vi "LSMcontroller_v57.vi"() -> ()   [LabVIEW 2015] (continued)
                              }
                            }
                          }
                        }
                        frame True {
                        }
                      }
                      n2928 = local read "sealtest 2"() -> (w5970:bool)
                      n2929 = Not(x=w5970) -> (.not. x?=w5969:bool)
                    }
                  }
                  frame #4 {
                    n2930 = call "tempconfigAO.vi"("command"="get") -> ("Temp Config out"=w6140:T27)  [unwired: 1 in]
                    n2931 = Unbundle By Name(w6140) -> ("AO"=w6139:refnum<k21>[], "E_AO"=w6138:errorcluster[])
                    n2932 = call "configuration.vi"("command"="get") -> ("config out"=w6121:T13)  [unwired: 2 in, 1 out]
                    n2933 = call "tempconfigAI.vi"("command"="get") -> ("Temp Config out"=w6127:T28)  [unwired: 1 in]
                    n2934 = Unbundle By Name(w6121) -> ("Device 1 sampleclock out"=w6118:tag, "Device 1 Starttrigger out"=w6117:tag)
                    n2935 = Unbundle By Name(w6127) -> ("AI"=w6128:refnum<k21>, "E_AI"=w6129:errorcluster)
                    n2936 = for {
                      tunnel: w6139 -> [w6144] mode=indexing
                      tunnel: w6138 -> [w6143] mode=indexing
                      tunnel: [w6142] -> w6134 mode=indexing
                      n2937 = call <vilib>:"DAQmx Stop Task.vi"("task/channels in"=w6144, "error in"=w6143) -> ("task out"=w6145:refnum<k21>, "error out"=w6146:errorcluster)  [unwired: 12 in]
                      n2938 = call <vilib>:"DAQmx Clear Task.vi"("task in"=w6145, "error in"=w6146) -> ("error out"=w6142:errorcluster)  [unwired: 13 in]
                    }
                    n2939 = call <vilib>:"DAQmx Stop Task.vi"("task/channels in"=w6128, "error in"=w6129) -> ("task out"=w6125:refnum<k21>, "error out"=w6124:errorcluster)  [unwired: 12 in]
                    n2940 = call <vilib>:"DAQmx Disconnect Terminals.vi"("source terminal"=tag "/Dev1/ai/SampleClock", "destination terminal"=w6118) -> ("error out"=w6115:errorcluster)  [unwired: 13 in]
                    n2941 = call <vilib>:"DAQmx Clear Task.vi"("task in"=w6125, "error in"=w6124) -> ("error out"=w6123:errorcluster)  [unwired: 13 in]
                    n2942 = call "tempconfigAO.vi"("command"="get") -> ("Temp Config out"=w6135:T27)  [unwired: 1 in]
                    n2943 = Bundle By Name(cluster=w6135, "E_AO"=w6134) -> (w6133:T27)
                    n2944 = call "tempconfigAI.vi"("command"="get") -> ("Temp Config out"=w6131:T28)  [unwired: 1 in]
                    n2945 = Bundle By Name(cluster=w6131, "E_AI"=w6123) -> (w6122:T28)
                    n2946 = call "tempconfigAO.vi"("Temp Config in"=w6133, "command"="set") -> ()  [unwired: 1 out]
                    n2947 = call <vilib>:"DAQmx Disconnect Terminals.vi"("source terminal"=tag "/Dev1/ai/StartTrigger", "destination terminal"=w6117, "error in"=w6115) -> ()  [unwired: 12 in, 1 out]
                    n2948 = call "tempconfigAI.vi"("Temp Config in"=w6122, "command"="set") -> ()  [unwired: 1 out]
                  }
                  frame #5 {
                    w6149 = T23 4 items=["no dialog", "OK message", "continue or stop message", "OK message + warnings", "continue/stop + warnings"] ("type of dialog (OK msg:1)")
                    n2949 = call "displayerrors.vi"() -> ("error IO"=w6148:errorcluster)
                    n2950 = call "zeropatch.vi"() -> ()  [unwired: 12 in]
                    n2951 = call <vilib>:"Simple Error Handler.vi"("type of dialog (OK msg:1)"=w6149, "error in (no error)"=w6148) -> ("error out"=w6147:errorcluster)  [unwired: 3 in, 4 out]
                    n2952 = call <vilib>:"Clear Errors.vi"("error in (no error)"=w6147) -> ()  [unwired: 5 in, 2 out]
                  }
                }
              }
            }
          }
          event "Current Clamp": Value Change {
            n2953 = event-data() -> ()  [unwired: 1 in, 6 out]
            n2954 = local read "Current Clamp"() -> (w6154:bool)
            n2955 = property on="Vholding (mV)" class="DigNum (strict)"("Caption.Text"="Ihold (pA)") -> ()  [unwired: 2 in, 2 out]
            n2956 = Not(x=w6154) -> (.not. x?=w6153:bool)
            n2957 = property on="Voltage Clamp" class="Bool (strict)"("Value"=w6153) -> ()  [unwired: 2 in, 2 out]
            n2958 = One Button Dialog(message="Have you switched the HEKA to CC and changed the external input cable?", button name ("OK")="Ok") -> ()  [unwired: 1 out]
          }
          event "Voltage Clamp": Value Change {
            n2959 = event-data() -> ()  [unwired: 1 in, 6 out]
            n2960 = local read "Voltage Clamp"() -> (w6159:bool)
            n2961 = Not(x=w6159) -> (.not. x?=w6158:bool)
            n2962 = property on="Current Clamp" class="Bool (strict)"("Value"=w6158) -> ()  [unwired: 2 in, 2 out]
            n2963 = One Button Dialog(message="Have you switched the HEKA to VC and changed the external input cable?", button name ("OK")="Ok") -> ()  [unwired: 1 out]
            n2964 = property on="Vholding (mV)" class="DigNum (strict)"("Caption.Text"="Vhold (mV)") -> ()  [unwired: 2 in, 2 out]
          }
          event "OCgain": Value Change {
            n2965 = event-data() -> ()  [unwired: 1 in, 6 out]
            n2966 = local read "OCgain"() -> (w6162:sgl)
            n2967 = Less?(x=w6162, y=0.3) -> (x < y?=w6160:bool)
            n2968 = case shown="True" w6160 {
              frame False {
                w6163 = 10.0 items=["0.1"=10.0, "10"=0.1] ("CC_ICgain")
                n2969 = local write "CC_ICgain"(w6163) -> ()
              }
              frame True {
                w6164 = 0.1 items=["0.1"=10.0, "10"=0.1] ("CC_ICgain")
                n2970 = local write "CC_ICgain"(w6164) -> ()
              }
            }
          }
          event "holdon": Value Change {
            n2971 = event-data() -> ()  [unwired: 1 in, 6 out]
            n2972 = stacked-sequence {
              frame #0 {
                n2973 = local read "Vholding (mV)"() -> (w6168:sgl)
                n2974 = local read "holdon"() -> (w6165:bool)
                n2975 = call "patchparameters.vi"("command"="get") -> ("Params out"=w6169:T15)  [unwired: 1 in]
                n2976 = Bundle By Name(cluster=w6169, "Vhold (mV)"=w6168, "holdon"=w6165) -> (w6166:T15)
                n2977 = call "patchparameters.vi"("Params in"=w6166, "command"="set") -> ()  [unwired: 1 out]
              }
              frame #1 {
                n2978 = call "zeropatch.vi"() -> ()  [unwired: 12 in]
              }
            }
          }
          event "Vholding (mV)": Value Change {
            n2979 = event-data() -> ()  [unwired: 1 in, 6 out]
            n2980 = local read "holdon"() -> (w6171:bool)
            n2981 = case shown="True" w6171 {
              frame False {
              }
              frame True {
                n2982 = stacked-sequence {
                  frame #0 {
                    n2983 = local read "Vholding (mV)"() -> (w6174:sgl)
                    n2984 = local read "holdon"() -> (w6175:bool)
                    n2985 = call "patchparameters.vi"("command"="get") -> ("Params out"=w6176:T15)  [unwired: 1 in]
                    n2986 = Bundle By Name(cluster=w6176, "Vhold (mV)"=w6174, "holdon"=w6175) -> (w6172:T15)
                    n2987 = call "patchparameters.vi"("Params in"=w6172, "command"="set") -> ()  [unwired: 1 out]
                  }
                  frame #1 {
                    n2988 = call "zeropatch.vi"() -> ()  [unwired: 12 in]
                  }
                }
              }
            }
          }
          event "readpatch": Value Change {
            n2989 = event-data() -> ("NewVal"=w6178:bool)  [unwired: 1 in, 5 out]
            n2990 = case shown="True" w6178 {
              frame False {
              }
              frame True {
                n2991 = stacked-sequence {
                  frame #0 {
                    n2992 = stacked-sequence {
                      frame #0 {
                        n2993 = call "2pparameters.vi"("command"="get") -> ("params out"=w6180:T12)  [unwired: 1 in]
                        n2994 = Unbundle By Name(w6180) -> ("autoshutter"=w6181:bool)
                        n2995 = case shown="True" w6181 {
                          frame False {
                          }
                          frame True {
                            n2996 = call "shuttercontrol.vi"("command"="close") -> ()  [unwired: 1 in, 1 out]
                          }
                        }
                      }
                      frame #1 {
                        n2997 = local read "Voltage Clamp"() -> (w6188:bool)
                        n2998 = local read "Current Clamp"() -> (w6189:bool)
                        n2999 = local read "Vholding (mV)"() -> (w6183:sgl)
                        n3000 = local read "CC_ICgain"() -> (w6187:dbl)
                        n3001 = local read "OCgain"() -> (w6184:sgl)
                        n3002 = call "patchparameters.vi"("command"="get") -> ("Params out"=w6191:T15)  [unwired: 1 in]
                        n3003 = Bundle By Name(cluster=w6191, "VC"=w6188, "CC"=w6189, "CC_icg (pA/mv)"=w6187, "VC_icg (mV/mV)"=10.0, "OCG (mV/pA)"=w6184, "OVG (mV/mV)"=0.1, "Vhold (mV)"=w6183) -> (w6190:T15)
                        n3004 = call "patchparameters.vi"("Params in"=w6190, "command"="set") -> ()  [unwired: 1 out]
                      }
                      frame #2 {
                        w6202 = 10123 items=["Finite Samples"=10178, "Continuous Samples"=10123, "Hardware Timed Single Point"=12522] ("sample mode")
                        n3005 = call "configuration.vi"("command"="get") -> ("config out"=w6197:T13)  [unwired: 2 in, 1 out]
                        n3006 = Unbundle By Name(w6197) -> ("Vp"=w6196:i32, "Ip"=w6195:i32)
                        n3007 = call "2pparameters.vi"("command"="get") -> ("params out"=w6205:T12)  [unwired: 1 in]
                        n3008 = Build Array(w6196, w6195) -> (w6194:i32[])
                        n3009 = Bundle By Name(cluster=w6205, "srate"=10000.0, "refreshbuffer"=500, "timeout"=10.0, "sample mode"=w6202, "aAI"=w6194) -> (w6203:T12)
                        n3010 = call "2pparameters.vi"("Params in"=w6203, "command"="set") -> ()  [unwired: 1 out]
                      }
                    }
                  }
                  frame #1 {
                    n3011 = while {
                      stop <- w6207 stop-if-true
                      n3012 = local read "readpatch"() -> (w6209:bool)
                      n3013 = case shown="True" w6209 {
                        frame False {
                        }
                        frame True {
                          n3014 = stacked-sequence {
                            frame #0 {
                              n3015 = local read "Vholding (mV)"() -> (w6212:sgl)
                              n3016 = local read "holdon"() -> (w6210:bool)
                              n3017 = call "patchparameters.vi"("command"="get") -> ("Params out"=w6213:T15)  [unwired: 1 in]
                              n3018 = Bundle By Name(cluster=w6213, "Vhold (mV)"=w6212, "holdon"=w6210) -> (w6211:T15)
                              n3019 = call "patchparameters.vi"("Params in"=w6211, "command"="set") -> ()  [unwired: 1 out]
                            }
                            frame #1 {
                              n3020 = call "zeropatch.vi"() -> ()  [unwired: 12 in]
                            }
                            frame #2 {
                              n3021 = call "prepAI_ttv2.vi"() -> ()  [unwired: 2 in, 1 out]
                            }
                            frame #3 {
                              n3022 = call "runAI_tt.vi"() -> ()  [unwired: 12 in]
                            }
                            frame #4 {
                              n3023 = call "collectAI_tt_V2.vi"() -> ()  [unwired: 4 in]
                            }
                            frame #5 {
                              n3024 = call "stoperaseAI_tt.vi"() -> ()  [unwired: 12 in]
                            }
                            frame #6 {
                              n3025 = call "tempconfigAI.vi"("command"="get") -> ("Temp Config out"=w6231:T28)  [unwired: 1 in]
                              n3026 = Unbundle By Name(w6231) -> ("header"=w6221:dbl[])
                              n3027 = call "allAI-temp.vi"("command"=enum16{"get", "set", "clear", "append"}."get") -> ("array out"=w6222:sgl[][])  [unwired: 3 in, 1 out]
                              n3028 = call "Unscaledtoscaled2D.vi"("Unscaled Data"=w6222, "Header Information"=w6221) -> ("Array"=w6220:sgl[][])  [unwired: 1 in]
                              n3029 = local read "OCgain"() -> (w6232:sgl)
                              n3030 = Index Array(array=w6220, index (row) #1=0 ("index (row)"), index (row) #2=1 ("index (row)")) -> (element #1=w6217:sgl[], element #2=w6216:sgl[])  [unwired: 2 in]
                              n3031 = Divide(x=w6217, y=w6232) -> (x/y=w6226:sgl[])
                              n3032 = Multiply(x=w6216, y=sgl 0.1) -> (x*y=w6225:sgl[])
                              n3033 = Build Array(w6226, w6225) -> (w6229:sgl[][])
                              n3034 = Multiply(x=w6229, y=sgl 1000.0) -> (x*y=w6224:sgl[][])
                              n3035 = local write "Patch readout"(w6224) -> ()
                            }
                          }
                        }
                      }
                      n3036 = local read "readpatch"() -> (w6208:bool)
                      n3037 = Not(x=w6208) -> (.not. x?=w6207:bool)
                    }
                  }
                  frame #2 {
                    w6235 = T23 4 items=["no dialog", "OK message", "continue or stop message", "OK message + warnings", "continue/stop + warnings"] ("type of dialog (OK msg:1)")
                    n3038 = call "displayerrors.vi"() -> ("error IO"=w6234:errorcluster)
                    n3039 = call <vilib>:"Simple Error Handler.vi"("type of dialog (OK msg:1)"=w6235, "error in (no error)"=w6234) -> ("error out"=w6233:errorcluster)  [unwired: 3 in, 4 out]
                    n3040 = call <vilib>:"Clear Errors.vi"("error in (no error)"=w6233) -> ()  [unwired: 5 in, 2 out]
                  }
                  frame #3 {
                    n3041 = call "zeropatch.vi"() -> ()  [unwired: 12 in]
                  }
                  frame #4 {
                    n3042 = disable-structure shown="Disabled" {
                      frame Disabled {
                        n3043 = local read item#-1() -> (w6241)
                        n3044 = local read item#-1() -> (w6240)
                        n3045 = local read item#-1() -> (w6237)
                        n3046 = local read item#-1() -> (w6239)
                        n3047 = local read item#-1() -> (w6238)
                        n3048 = local read item#-1() -> (w6236)
                        n3049 = call "waveformparamsv2.vi"("command"="get") -> ("Params out"=w6243:T24)  [unwired: 1 in]
                        n3050 = Bundle By Name(cluster=w6243, "patch"=w6241, "laserAO"=w6240, "shutter"=w6239, "488"=w6238, "532"=w6237, "640"=w6236) -> (w6242:T24)
                        n3051 = call "waveformparamsv2.vi"("Params in"=w6242, "command"="set") -> ()  [unwired: 1 out]
                      }
                      frame Enabled {
                      }
                    }
                  }
                  frame #5 {
                    n3052 = call "2pparameters.vi"("command"="get") -> ("params out"=w6247:T12)  [unwired: 1 in]
                    n3053 = Unbundle By Name(w6247) -> ("autoshutter"=w6248:bool)
                    n3054 = case shown="True" w6248 {
                      frame False {
                      }
                      frame True {
                        n3055 = call "shuttercontrol.vi"("command"="close") -> ()  [unwired: 1 in, 1 out]
                      }
                    }
                  }
                }
              }
            }
          }
          event "AI channels": Value Change {
            n3056 = event-data() -> ()  [unwired: 1 in, 6 out]
            n3057 = local read "CI channels"() -> (w6257:i32[])
            n3058 = local read "AI channels"() -> (w6258:i32[])
            n3059 = call "configuration.vi"("command"="get") -> ("config out"=w6251:T13)  [unwired: 2 in, 1 out]
            n3060 = Unbundle By Name(w6251) -> ("CI names"=w6252:string[], "AI names"=w6253:string[])
            n3061 = for {
              tunnel: w6257 -> [w6263] mode=indexing
              tunnel: w6252 -> [w6264]
              tunnel: [w6262] -> w6254 mode=indexing
              n3062 = Index Array(array=w6264, index=w6263) -> (element=w6262:string)
            }
            n3063 = for {
              tunnel: w6258 -> [w6260] mode=indexing
              tunnel: w6253 -> [w6261]
              tunnel: [w6259] -> w6255 mode=indexing
              n3064 = Index Array(array=w6261, index=w6260) -> (element=w6259:string)
            }
            n3065 = Build Array (concatenate)(w6254, w6255) -> (w6256:string[])
            n3066 = property on="image1list" class="Ring (strict)"("Strings []"=w6256) -> ()  [unwired: 2 in, 2 out]
            n3067 = property on="image2list" class="Ring (strict)"("Strings []"=w6256) -> ()  [unwired: 2 in, 2 out]
          }
          event "CI channels": Value Change {
            n3068 = event-data() -> ()  [unwired: 1 in, 6 out]
            n3069 = local read "CI channels"() -> (w6272:i32[])
            n3070 = local read "AI channels"() -> (w6273:i32[])
            n3071 = call "configuration.vi"("command"="get") -> ("config out"=w6266:T13)  [unwired: 2 in, 1 out]
            n3072 = Unbundle By Name(w6266) -> ("CI names"=w6267:string[], "AI names"=w6268:string[])
            n3073 = for {
              tunnel: w6272 -> [w6278] mode=indexing
              tunnel: w6267 -> [w6279]
              tunnel: [w6277] -> w6269 mode=indexing
              n3074 = Index Array(array=w6279, index=w6278) -> (element=w6277:string)
            }
            n3075 = for {
              tunnel: w6273 -> [w6275] mode=indexing
              tunnel: w6268 -> [w6276]
              tunnel: [w6274] -> w6270 mode=indexing
              n3076 = Index Array(array=w6276, index=w6275) -> (element=w6274:string)
            }
            n3077 = Build Array (concatenate)(w6269, w6270) -> (w6271:string[])
            n3078 = property on="image1list" class="Ring (strict)"("Strings []"=w6271) -> ()  [unwired: 2 in, 2 out]
            n3079 = property on="image2list" class="Ring (strict)"("Strings []"=w6271) -> ()  [unwired: 2 in, 2 out]
          }
          event "setdatdir": Value Change {
            n3080 = event-data() -> ()  [unwired: 1 in, 5 out]
            n3081 = case shown="True" "setdatdir" {
              frame False {
              }
              frame True {
                n3082 = stacked-sequence {
                  frame #0 {
                    n3083 = local read "data dir"() -> (w6281:path)
                    n3084 = call "File Dialog"("start path"=w6281, "prompt"="Please select data directory...") -> ("selected path"=w6283:path, "cancelled"=w6282:bool, "error out"=w6284:errorcluster)  [unwired: 10 in, 1 out]
                    n3085 = case shown="False" w6282 {
                      tunnel: w6283 -> [w6292 _]
                      tunnel: w6284 -> [w6289 w6295]
                      tunnel: [w6287 w6295] -> w6286
                      frame False {
                        n3086 = local write "data dir"(w6292) -> ()
                        n3087 = call "configuration.vi"("error in"=w6289, "command"="get") -> ("Error out"=w6288:errorcluster, "config out"=w6294:T13)  [unwired: 1 in]
                        n3088 = Bundle By Name(cluster=w6294, "master data dir"=w6292) -> (w6293:T13)
                        n3089 = call "configuration.vi"("error in"=w6288, "config in"=w6293, "command"="set") -> ("Error out"=w6287:errorcluster)  [unwired: 1 out]
                      }
                      frame True {
                      }
                    }
                    n3090 = local write "status"(w6286) -> ()
                  }
                  frame #1 {
                    n3091 = property on="setdatdir" class="Bool (strict)"("Value"=FALSE ("setdatdir")) -> ()  [unwired: 2 in, 2 out]
                  }
                }
              }
            }
          }
          event "Shutter": Value Change {
            n3092 = event-data() -> ()  [unwired: 1 in, 5 out]
            n3093 = case shown="False" "Shutter" {
              frame False {
                n3094 = call "shuttercontrol.vi"("command"="close") -> ()  [unwired: 1 in, 1 out]
              }
              frame True {
                n3095 = call "shuttercontrol.vi"("command"="open") -> ()  [unwired: 1 in, 1 out]
              }
            }
          }
          event "ROI": Value Change {
            n3096 = event-data() -> ()  [unwired: 1 in, 5 out]
            n3097 = local read "ROI"() -> (w6300:bool)
            n3098 = case shown="True" w6300 {
              frame False {
              }
              frame True {
                n3099 = stacked-sequence {
                  frame #0 {
                    n3100 = local read "Square pixels"() -> (w6317:bool)
                    n3101 = local read "square matrix"() -> (w6316:bool)
                    n3102 = local read "Vx-max ref"() -> (w6322:dbl)
                    n3103 = local read "Vx-min ref"() -> (w6321:dbl)
                    n3104 = local read "Vy-min ref"() -> (w6318:dbl)
                    n3105 = local read "ypixels ref"() -> (w6320:i32)
                    n3106 = local read "Vy-max ref"() -> (w6319:dbl)
                    n3107 = local read "xpixels ref"() -> (w6323:i32)
                    n3108 = local read "Angle ref"() -> (w6315:dbl)
                    n3109 = local read "Colormap"() -> (w6324:i32)
                    n3110 = call "2pparameters.vi"("command"="get") -> ("params out"=w6327:T12)  [unwired: 1 in]
                    n3111 = Bundle By Name(cluster=w6327, "Xpixels Img"=w6323, "Vx-min Img"=w6321, "VX-max Img"=w6322, "Ypixels Img"=w6320, "Vy-min Img"=w6318, "Vy-max Img"=w6319, "Colormap"=w6324, "square pixels"=w6317, "square matrix"=w6316, "Angle Img"=w6315) -> (w6326:T12)
                    n3112 = call "2pparameters.vi"("Params in"=w6326, "command"="set") -> ()  [unwired: 1 out]
                    n3113 = local read "Vx-max draw"() -> (w6307:dbl)
                    n3114 = local read "Angle drawing"() -> (w6314:dbl)
                    n3115 = local read "Vx-min draw"() -> (w6308:dbl)
                    n3116 = local read "Vy-min draw"() -> (w6311:dbl)
                    n3117 = local read "ypixels draw"() -> (w6309:dbl)
                    n3118 = local read "Vy-max draw"() -> (w6310:dbl)
                    n3119 = local read "Square pixels"() -> (w6312:bool)
                    n3120 = local read "square matrix"() -> (w6313:bool)
                    n3121 = local read "xpixels draw"() -> (w6306:dbl)
                    n3122 = local read "Colormap"() -> (w6305:i32)
                    n3123 = call "2pparameters.vi"("command"="get") -> ("params out"=w6302:T12)  [unwired: 1 in]
                    n3124 = Bundle By Name(cluster=w6302, "Xpixels"=w6306, "Vxminref"=w6308, "Vxmaxref"=w6307, "Ypixels"=w6309, "Vyminref"=w6311, "Vymaxref"=w6310, "Colormap"=w6305, "square pixels"=w6312, "square matrix"=w6313, "Angle draw"=w6314) -> (w6303:T12)
                    n3125 = call "2pparameters.vi"("Params in"=w6303, "command"="set") -> ()  [unwired: 1 out]
                  }
                  frame #1 {
                    n3126 = Current VI's Path() -> (path=w6338:path)
                    n3127 = Strip Path(path=w6338) -> (stripped path=w6339:path)  [unwired: 1 out]
                    n3128 = Build Path(base path=w6339, name or relative path="subVIs\\Image\\SetROI_v3.vi") -> (appended path=w6337:path)
                    n3129 = call <vilib>:"Set Busy.vi"() -> ("error out"=w6335:errorcluster)  [unwired: 10 in, 1 out]
                    n3130 = Open VI Reference(type specifier VI Refnum (for type only)=refnum<vi> refnum, vi path=w6337, error in (no error)=w6335) -> (vi reference=w6333:refnum<vi>, error out=w6331:errorcluster)  [unwired: 3 in]
                    n3131 = call-by-ref "?"(reference=w6333, error in=w6331) -> (reference out=w6332:refnum<vi>, error out=w6330:errorcluster)  [unwired: 1 in]
                    n3132 = Close Reference(reference=w6332, error in (no error)=w6330) -> (error out=w6334:errorcluster)
                    n3133 = call <vilib>:"Unset Busy.vi"("error in (no error)"=w6334) -> ()  [unwired: 10 in, 1 out]
                    n3134 = local write "status"(w6334) -> ()
                  }
                  frame #2 {
                    n3135 = call "2pparameters.vi"("command"="get") -> ("params out"=w6364:T12)  [unwired: 1 in]
                    n3136 = Unbundle By Name(w6364) -> ("Xpixels Img"=w6363:i32, "Vx-min Img"=w6362:dbl, "VX-max Img"=w6361:dbl, "Ypixels Img"=w6360:i32, "Vy-min Img"=w6359:dbl, "Vy-max Img"=w6358:dbl, "Colormap"=w6357:u16, "square pixels"=w6356:bool, "square matrix"=w6355:bool, "Angle Img"=w6354:dbl, "Drawing Mode"=w6353:u16)
                    n3137 = local write "xpixels ref"(w6363) -> ()
                    n3138 = local write "Vx-min ref"(w6362) -> ()
                    n3139 = local write "Vx-max ref"(w6361) -> ()
                    n3140 = local write "ypixels ref"(w6360) -> ()
                    n3141 = local write "Vy-min ref"(w6359) -> ()
                    n3142 = local write "Vy-max ref"(w6358) -> ()
                    n3143 = local write "Colormap"(w6357) -> ()
                    n3144 = local write "Square pixels"(w6356) -> ()
                    n3145 = local write "square matrix"(w6355) -> ()
                    n3146 = local write "Angle ref"(w6354) -> ()
                    n3147 = local write "ROI Type"(w6353) -> ()
                    n3148 = call "2pparameters.vi"("command"="get") -> ("params out"=w6347:T12)  [unwired: 1 in]
                    n3149 = Unbundle By Name(w6347) -> ("Xpixels"=w6341:i32, "Vxminref"=w6345:dbl, "Vxmaxref"=w6344:dbl, "Ypixels"=w6340:i32, "Vyminref"=w6343:dbl, "Vymaxref"=w6342:dbl, "Colormap"=w6348:u16, "square pixels"=w6349:bool, "square matrix"=w6350:bool, "Angle draw"=w6351:dbl, "Drawing Mode"=w6352:u16)
                    n3150 = local write "Vy-max draw"(w6342) -> ()
                    n3151 = local write "Angle drawing"(w6351) -> ()
                    n3152 = local write "Colormap"(w6348) -> ()
                    n3153 = local write "Square pixels"(w6349) -> ()
                    n3154 = local write "square matrix"(w6350) -> ()
                    n3155 = local write "ROI Type"(w6352) -> ()
                    n3156 = local write "xpixels draw"(w6341) -> ()
                    n3157 = local write "ypixels draw"(w6340) -> ()
                    n3158 = local write "Vx-min draw"(w6345) -> ()
                    n3159 = local write "Vx-max draw"(w6344) -> ()
                    n3160 = local write "Vy-min draw"(w6343) -> ()
                  }
                  frame #3 {
                    n3161 = property on="ROI" class="Bool (strict)"("Val(Sgnl)"=FALSE ("x/y scan")) -> ()  [unwired: 2 in, 2 out]
                  }
                }
              }
            }
          }
          event "Xdattype": Value Change {
            n3162 = event-data() -> ()  [unwired: 1 in, 1 out]
            n3163 = case shown="True" "Xdattype" {
              frame False {
              }
              frame True {
                n3164 = stacked-sequence {
                  frame #0 {
                    n3165 = Current VI's Path() -> (path=w6377:path)
                    n3166 = Strip Path(path=w6377) -> (stripped path=w6378:path)  [unwired: 1 out]
                    n3167 = Build Path(base path=w6378, name or relative path="subVIs\\Misc\\Changedataconfig.vi") -> (appended path=w6376:path)
                    n3168 = call <vilib>:"Set Busy.vi"() -> ("error out"=w6374:errorcluster)  [unwired: 10 in, 1 out]
                    n3169 = Open VI Reference(type specifier VI Refnum (for type only)=refnum<vi> refnum, vi path=w6376, error in (no error)=w6374) -> (vi reference=w6369:refnum<vi>, error out=w6371:errorcluster)  [unwired: 3 in]
                    n3170 = call-by-ref "?"(reference=w6369, error in=w6371) -> (reference out=w6373:refnum<vi>, error out=w6372:errorcluster)  [unwired: 12 in]
                    n3171 = Close Reference(reference=w6373, error in (no error)=w6372) -> (error out=w6368:errorcluster)
                    "status" <- w6368
                    n3172 = call <vilib>:"Unset Busy.vi"("error in (no error)"=w6368) -> ()  [unwired: 10 in, 1 out]
                  }
                  frame #1 {
                    n3173 = property on="Xdattype" class="Bool (strict)"("Val(Sgnl)"=FALSE ("x/y scan")) -> ()  [unwired: 2 in, 2 out]
                  }
                }
              }
            }
          }
          event "XautoOD": Value Change {
            n3174 = event-data() -> ()  [unwired: 1 in, 1 out]
            n3175 = case shown="True" "XautoOD" {
              frame False {
              }
              frame True {
                n3176 = stacked-sequence {
                  frame #0 {
                    n3177 = Current VI's Path() -> (path=w6390:path)
                    n3178 = Strip Path(path=w6390) -> (stripped path=w6391:path)  [unwired: 1 out]
                    n3179 = Build Path(base path=w6391, name or relative path="subVIs\\Misc\\ChangeautoODs.vi") -> (appended path=w6389:path)
                    n3180 = call <vilib>:"Set Busy.vi"() -> ("error out"=w6387:errorcluster)  [unwired: 10 in, 1 out]
                    n3181 = Open VI Reference(type specifier VI Refnum (for type only)=refnum<vi> refnum, vi path=w6389, error in (no error)=w6387) -> (vi reference=w6382:refnum<vi>, error out=w6384:errorcluster)  [unwired: 3 in]
                    n3182 = call-by-ref "?"(reference=w6382, error in=w6384) -> (reference out=w6386:refnum<vi>, error out=w6385:errorcluster)  [unwired: 12 in]
                    n3183 = Close Reference(reference=w6386, error in (no error)=w6385) -> (error out=w6381:errorcluster)
                    "status 2" <- w6381
                    n3184 = call <vilib>:"Unset Busy.vi"("error in (no error)"=w6381) -> ()  [unwired: 10 in, 1 out]
                  }
                  frame #1 {
                    n3185 = property on="XautoOD" class="Bool (strict)"("Val(Sgnl)"=FALSE ("x/y scan")) -> ()  [unwired: 2 in, 2 out]
                  }
                }
              }
            }
          }
          event "SetMan": Value Change {
            n3186 = event-data() -> ()  [unwired: 1 in, 1 out]
            n3187 = case shown="True" "SetMan" {
              frame False {
              }
              frame True {
                n3188 = stacked-sequence {
                  frame #0 {
                    w6394 = u16 0 items=["Rectangle", "Circle", "Freeform Boundary", "Freeform Interior"] ("ROI Type")
                    n3189 = local write "ROI Type"(w6394) -> ()
                    n3190 = local read "Square pixels"() -> (w6400:bool)
                    n3191 = case shown="True" w6400 {
                      frame False {
                        n3192 = local read "square matrix"() -> (w6401:bool)
                        n3193 = case shown="False" w6401 {
                          frame False {
                            "ypixels ref" <- "ypixels"
                            "xpixels ref" <- "xpixels"
                          }
                          frame True {
                            n3194 = local read "xpixels"() -> (w6406:i32)
                            n3195 = local read "ypixels"() -> (w6405:i32)
                            n3196 = Max & Min(x=w6406, y=w6405) -> (max(x,y)=w6404:i32)  [unwired: 1 out]
                            n3197 = local write "xpixels ref"(w6404) -> ()
                            n3198 = local write "ypixels ref"(w6404) -> ()
                          }
                        }
                      }
                      frame True {
                        n3199 = local read "square matrix"() -> (w6407:bool)
                        n3200 = case shown="False" w6407 {
                          frame False {
                            n3201 = local read "Vxmax"() -> (w6421:dbl)
                            n3202 = local read "Vx-min"() -> (w6420:dbl)
                            n3203 = local read "Vy-max"() -> (w6416:dbl)
                            n3204 = local read "Vy-min"() -> (w6417:dbl)
                            n3205 = Subtract(x=w6416, y=w6417) -> (x-y=w6418:dbl)
                            n3206 = Subtract(x=w6421, y=w6420) -> (x-y=w6419:dbl)
                            n3207 = Absolute Value(x=w6418) -> (abs(x)=w6409:dbl)
                            n3208 = Absolute Value(x=w6419) -> (abs(x)=w6410:dbl)
                            n3209 = Divide(x=w6410, y=w6409) -> (x/y=w6415:dbl)
                            n3210 = Greater Or Equal?(x=w6410, y=w6409) -> (x >= y?=w6408:bool)
                            n3211 = local read "xpixels"() -> (w6414:i32)
                            n3212 = local read "ypixels"() -> (w6411:i32)
                            n3213 = case shown="False" w6408 {
                              tunnel: w6415 -> [w6426 w6429]
                              tunnel: w6414 -> [w6423 _]
                              tunnel: [w6423 w6428] -> w6413
                              tunnel: [w6422 w6427] -> w6412
                              tunnel: w6411 -> [_ w6427]
                              frame False {
                                n3214 = To Double Precision Float(number=w6423) -> (double precision float=w6425:dbl)
                                n3215 = Divide(x=w6425, y=w6426) -> (x/y=w6424:dbl)
                                n3216 = To Long Integer(number=w6424) -> (32bit integer=w6422:i32)
                              }
                              frame True {
                                n3217 = To Double Precision Float(number=w6427) -> (double precision float=w6431:dbl)
                                n3218 = Multiply(x=w6431, y=w6429) -> (x*y=w6430:dbl)
                                n3219 = To Long Integer(number=w6430) -> (32bit integer=w6428:i32)
                              }
                            }
                            n3220 = local write "ypixels ref"(w6412) -> ()
                            n3221 = local write "xpixels ref"(w6413) -> ()
                          }
                          frame True {
                          }
                        }
                      }
                    }
                    "Vx-max ref" <- "Vxmax"
                    "Vx-min ref" <- "Vx-min"
                    "Vy-max ref" <- "Vy-max"
                    "Vy-min ref" <- "Vy-min"
                    "Angle ref" <- "Angle"
                  }
                  frame #1 {
                    n3222 = property on="SetMan" class="Bool (strict)"("Val(Sgnl)"=FALSE ("Value (Signaling)")) -> ()  [unwired: 2 in, 2 out]
                  }
                }
              }
            }
          }
          event "SetMan 2": Value Change {
            n3223 = event-data() -> ()  [unwired: 1 in, 1 out]
            n3224 = case shown="True" "SetMan 2" {
              frame False {
              }
              frame True {
                n3225 = stacked-sequence {
                  frame #0 {
                    n3226 = local write "Vx-ref"("Vx") -> ()
                    n3227 = local write "Vy-ref"("Vy") -> ()
                  }
                  frame #1 {
                    n3228 = property on="SetMan 2" class="Bool (strict)"("Val(Sgnl)"=FALSE ("Value (Signaling)")) -> ()  [unwired: 2 in, 2 out]
                  }
                }
              }
            }
          }
          event "Reset Coords": Value Change {
            n3229 = event-data() -> ("NewVal"=w6437:bool)  [unwired: 1 in, 5 out]
            n3230 = case shown="True" w6437 {
              frame False {
              }
              frame True {
                n3231 = stacked-sequence {
                  frame #0 {
                    n3232 = local write "xpixels"(256 ("xpixels")) -> ()
                    n3233 = local write "ypixels"(256 ("ypixels")) -> ()
                    n3234 = local write "Vxmax"(9.0 ("Vx-max")) -> ()
                    n3235 = local write "Vx-min"(-9.0 ("Vx-min")) -> ()
                    n3236 = local write "Vy-max"(9.0 ("Vy-max")) -> ()
                    n3237 = local write "Vy-min"(-9.0 ("Vy-min")) -> ()
                    n3238 = local write "Angle"(0.0 ("Angle")) -> ()
                  }
                  frame #1 {
                    n3239 = property on="Reset Coords" class="Bool (strict)"("Value"=FALSE ("TROI")) -> ()  [unwired: 2 in, 2 out]
                  }
                }
              }
            }
          }
          event "TROI": Value Change {
            n3240 = event-data() -> ()  [unwired: 1 in, 1 out]
            n3241 = case shown="True" "TROI" {
              frame False {
              }
              frame True {
                n3242 = stacked-sequence {
                  frame #0 {
                    n3243 = local read "Vy-min ref"() -> (w6451:dbl)
                    n3244 = local read "Vy-max ref"() -> (w6450:dbl)
                    n3245 = local read "Vx-max ref"() -> (w6448:dbl)
                    n3246 = local read "Vx-min ref"() -> (w6449:dbl)
                    n3247 = local read "ypixels ref"() -> (w6453:i32)
                    n3248 = local read "xpixels ref"() -> (w6452:i32)
                    n3249 = local read "Angle ref"() -> (w6447:dbl)
                    n3250 = local write "Angle"(w6447) -> ()
                    n3251 = local write "xpixels"(w6452) -> ()
                    n3252 = local write "Vy-min"(w6451) -> ()
                    n3253 = local write "Vy-max"(w6450) -> ()
                    n3254 = local write "Vx-min"(w6449) -> ()
                    n3255 = local write "ypixels"(w6453) -> ()
                    n3256 = local write "Vxmax"(w6448) -> ()
                  }
                  frame #1 {
                    n3257 = property on="TROI" class="Bool (strict)"("Value"=FALSE ("TROI")) -> ()  [unwired: 2 in, 2 out]
                  }
                }
              }
            }
          }
          event "TROI 2": Value Change {
            n3258 = event-data() -> ()  [unwired: 1 in, 1 out]
            n3259 = case shown="True" "TROI 2" {
              frame False {
              }
              frame True {
                n3260 = stacked-sequence {
                  frame #0 {
                    n3261 = local read "Vx-ref"() -> (w6456:dbl)
                    n3262 = local read "Vy-ref"() -> (w6457:dbl)
                    n3263 = local write "Vx"(w6456) -> ()
                    n3264 = local write "Vy"(w6457) -> ()
                  }
                  frame #1 {
                    n3265 = property on="TROI 2" class="Bool (strict)"("Value"=FALSE ("TROI")) -> ()  [unwired: 2 in, 2 out]
                  }
                }
              }
            }
          }
          event "Square pixels": Value Change {
            n3266 = event-data() -> ()  [unwired: 1 in, 1 out]
            n3267 = case shown="True" "Square pixels" {
              frame False {
              }
              frame True {
                n3268 = property on="square matrix" class="Bool (strict)"("Value"=FALSE ("square matrix")) -> ()  [unwired: 2 in, 2 out]
                n3269 = property on="Square pixels" class="Bool (strict)"("Value"=TRUE ("square matrix")) -> ()  [unwired: 2 in, 2 out]
              }
            }
          }
          event "square matrix": Value Change {
            n3270 = event-data() -> ()  [unwired: 1 in, 1 out]
            n3271 = case shown="True" "square matrix" {
              frame False {
              }
              frame True {
                n3272 = property on="square matrix" class="Bool (strict)"("Value"=TRUE ("square matrix")) -> ()  [unwired: 2 in, 2 out]
                n3273 = property on="Square pixels" class="Bool (strict)"("Value"=FALSE ("square matrix")) -> ()  [unwired: 2 in, 2 out]
              }
            }
          }
          event "up", "downright", "down", "downleft", "right", "left", "upright", "upleft": Value Change {
            n3274 = event-data() -> ()  [unwired: 1 in, 6 out]
            n3275 = local read "downright"() -> (w6470:bool)
            n3276 = local read "downleft"() -> (w6472:bool)
            n3277 = local read "upright"() -> (w6468:bool)
            n3278 = local read "upleft"() -> (w6466:bool)
            n3279 = local read "down"() -> (w6471:bool)
            n3280 = local read "right"() -> (w6469:bool)
            n3281 = local read "left"() -> (w6473:bool)
            n3282 = local read "up"() -> (w6467:bool)
            n3283 = Compound Arithmetic op=OR(w6466, w6467, w6468, w6469, w6470, w6471, w6472, w6473) -> (w6465:bool)
            n3284 = case shown="True" w6465 {
              frame False {
              }
              frame True {
                n3285 = stacked-sequence {
                  frame #0 {
                    n3286 = local read "downright"() -> (w6475:bool)
                    n3287 = local read "downleft"() -> (w6477:bool)
                    n3288 = local read "BigSmall"() -> (w6474:bool)
                    n3289 = local read "upright"() -> (w6479:bool)
                    n3290 = local read "upleft"() -> (w6482:bool)
                    n3291 = local read "down"() -> (w6478:bool)
                    n3292 = local read "right"() -> (w6480:bool)
                    n3293 = local read "left"() -> (w6476:bool)
                    n3294 = local read "up"() -> (w6481:bool)
                    n3295 = call "movestageparams.vi"("command"="get") -> ("Params out"=w6485:T22)  [unwired: 1 in]
                    n3296 = Bundle By Name(cluster=w6485, "upleft"=w6482, "up"=w6481, "upright"=w6479, "right"=w6480, "downright"=w6475, "down"=w6478, "downleft"=w6477, "left"=w6476, "Bigsmall"=w6474) -> (w6486:T22)
                    n3297 = call "movestageparams.vi"("Params in"=w6486, "command"="set") -> ()  [unwired: 1 out]
                  }
                  frame #1 {
                    n3298 = disable-structure shown="Disabled" {
                      frame Disabled {
                        n3299 = call "configuration.vi"("command"="get") -> ("config out"=w6489:T13)  [unwired: 2 in, 1 out]
                        n3300 = in-place {
                          n3301 = in-place-cluster #45(w6489) -> ()  [unwired: 2 out]
                          n3302 = in-place-cluster #45("StageL"="StageL", "StageS"="StageS") -> (w6487:T13)
                        }
                        n3303 = call "configuration.vi"("config in"=w6487, "command"="set") -> ()  [unwired: 1 in, 2 out]
                      }
                      frame Enabled {
                      }
                    }
                  }
                  frame #2 {
                    n3304 = call "movestage.vi"() -> ()  [unwired: 12 in]
                  }
                  frame #3 {
                    w6493 = FALSE ("OK Button")
                    w6494 = FALSE ("OK Button")
                    n3305 = property on="down" class="Bool (strict)"("Value"=w6494) -> ()  [unwired: 2 in, 2 out]
                    n3306 = property on="up" class="Bool (strict)"("Value"=w6494) -> ()  [unwired: 2 in, 2 out]
                    n3307 = property on="right" class="Bool (strict)"("Value"=w6494) -> ()  [unwired: 2 in, 2 out]
                    n3308 = property on="left" class="Bool (strict)"("Value"=w6494) -> ()  [unwired: 2 in, 2 out]
                    n3309 = property on="upright" class="Bool (strict)"("Value"=w6493) -> ()  [unwired: 2 in, 2 out]
                    n3310 = property on="downleft" class="Bool (strict)"("Value"=w6493) -> ()  [unwired: 2 in, 2 out]
                    n3311 = property on="downright" class="Bool (strict)"("Value"=w6493) -> ()  [unwired: 2 in, 2 out]
                    n3312 = property on="upleft" class="Bool (strict)"("Value"=w6493) -> ()  [unwired: 2 in, 2 out]
                  }
                }
              }
            }
          }
          event "finite samples": Value Change {
            n3313 = event-data() -> ("NewVal"=w6495:bool)  [unwired: 1 in]
            n3314 = flat-sequence {
              tunnel: w6495 -> [w6496]
              frame #0 {
                n3315 = case shown="True" w6496 {
                  frame False {
                    w6497 = FALSE ("wavdet")
                    n3316 = property on="continuous" class="Bool (strict)"("Value"=TRUE ("continuous for display")) -> ()  [unwired: 2 in, 2 out]
                    n3317 = property on="wavdet" class="Bool (strict)"("Value"=w6497) -> ()  [unwired: 2 in, 2 out]
                    n3318 = property on="save\ndata" class="Bool (strict)"("Value"=w6497) -> ()  [unwired: 2 in, 2 out]
                    n3319 = property on="# of frames" class="DigNum (strict)"("DisabledEnum"=T8."Disabled and Grayed Out" ("Disabled")) -> ()  [unwired: 2 in, 2 out]
                    n3320 = property on="save\ndata" class="Bool (strict)"("DisabledEnum"=T8."Disabled and Grayed Out" ("Disabled")) -> ()  [unwired: 2 in, 2 out]
                    "Save tab" <- enum32{"withsave", "withoutsave"}."withsave" ("Save tab")
                  }
                  frame True {
                    w6504 = FALSE ("continuous for display")
                    n3321 = property on="continuous" class="Bool (strict)"("Value"=w6504) -> ()  [unwired: 2 in, 2 out]
                    n3322 = property on="wavdet" class="Bool (strict)"("Value"=w6504) -> ()  [unwired: 2 in, 2 out]
                    n3323 = local write "Save tab"(enum32{"withsave", "withoutsave"}."withsave" ("Save tab")) -> ()
                    n3324 = property on="save\ndata" class="Bool (strict)"("DisabledEnum"=T8."Enabled" ("Disabled")) -> ()  [unwired: 2 in, 2 out]
                    n3325 = property on="save\ndata" class="Bool (strict)"("Value"=TRUE ("save\ndata")) -> ()  [unwired: 2 in, 2 out]
                    n3326 = property on="# of frames" class="DigNum (strict)"("DisabledEnum"=T8."Enabled" ("Disabled")) -> ()  [unwired: 2 in, 2 out]
                  }
                }
              }
              frame #1 {
                n3327 = local read "finite samples"() -> (w6513:bool)
                n3328 = local read "continuous"() -> (w6512:bool)
                n3329 = local read "wavdet"() -> (w6511:bool)
                n3330 = call "2pparameters.vi"("command"="get") -> ("params out"=w6507:T12)  [unwired: 1 in]
                n3331 = Bundle By Name(cluster=w6507, "finite"=w6513, "cont"=w6512, "wavdet"=w6511) -> (w6510:T12)
                n3332 = call "2pparameters.vi"("Params in"=w6510, "command"="set") -> ()  [unwired: 1 out]
              }
            }
          }
          event "continuous": Value Change {
            n3333 = event-data() -> ("NewVal"=w6514:bool)  [unwired: 1 in]
            n3334 = flat-sequence {
              tunnel: w6514 -> [w6515]
              frame #0 {
                n3335 = case shown="True" w6515 {
                  frame False {
                    n3336 = property on="finite samples" class="Bool (strict)"("Value"=TRUE ("finite samples for recording")) -> ()  [unwired: 2 in, 2 out]
                    n3337 = property on="save\ndata" class="Bool (strict)"("Value"=TRUE ("save\ndata")) -> ()  [unwired: 2 in, 2 out]
                    n3338 = property on="wavdet" class="Bool (strict)"("Value"=FALSE ("wavdet")) -> ()  [unwired: 2 in, 2 out]
                    n3339 = local write "Save tab"(enum32{"withsave", "withoutsave"}."withsave" ("Save tab")) -> ()
                    n3340 = property on="# of frames" class="DigNum (strict)"("DisabledEnum"=T8."Enabled" ("Disabled")) -> ()  [unwired: 2 in, 2 out]
                    n3341 = property on="save\ndata" class="Bool (strict)"("DisabledEnum"=T8."Enabled" ("Disabled")) -> ()  [unwired: 2 in, 2 out]
                  }
                  frame True {
                    w6522 = FALSE ("finite samples for recording")
                    n3342 = property on="finite samples" class="Bool (strict)"("Value"=w6522) -> ()  [unwired: 2 in, 2 out]
                    n3343 = property on="wavdet" class="Bool (strict)"("Value"=w6522) -> ()  [unwired: 2 in, 2 out]
                    n3344 = property on="save\ndata" class="Bool (strict)"("Value"=w6522) -> ()  [unwired: 2 in, 2 out]
                    n3345 = local write "Save tab"(enum32{"withsave", "withoutsave"}."withsave" ("Save tab")) -> ()
                    n3346 = property on="# of frames" class="DigNum (strict)"("DisabledEnum"=T8."Disabled and Grayed Out" ("Disabled")) -> ()  [unwired: 2 in, 2 out]
                    n3347 = property on="save\ndata" class="Bool (strict)"("DisabledEnum"=T8."Disabled and Grayed Out" ("Disabled")) -> ()  [unwired: 2 in, 2 out]
                  }
                }
              }
              frame #1 {
                n3348 = local read "finite samples"() -> (w6532:bool)
                n3349 = local read "continuous"() -> (w6531:bool)
                n3350 = local read "wavdet"() -> (w6530:bool)
                n3351 = call "2pparameters.vi"("command"="get") -> ("params out"=w6526:T12)  [unwired: 1 in]
                n3352 = Bundle By Name(cluster=w6526, "finite"=w6532, "cont"=w6531, "wavdet"=w6530) -> (w6529:T12)
                n3353 = call "2pparameters.vi"("Params in"=w6529, "command"="set") -> ()  [unwired: 1 out]
              }
            }
          }
          event "wavdet": Value Change {
            n3354 = event-data() -> ("NewVal"=w6533:bool)  [unwired: 1 in]
            n3355 = flat-sequence {
              tunnel: w6533 -> [w6534]
              frame #0 {
                n3356 = case shown="False" w6534 {
                  frame False {
                    n3357 = property on="finite samples" class="Bool (strict)"("Value"=TRUE ("finite samples for recording")) -> ()  [unwired: 2 in, 2 out]
                    n3358 = property on="continuous" class="Bool (strict)"("Value"=FALSE ("continuous")) -> ()  [unwired: 2 in, 2 out]
                    n3359 = local write "Save tab"(enum32{"withsave", "withoutsave"}."withsave" ("Save tab")) -> ()
                    n3360 = property on="save\ndata" class="Bool (strict)"("DisabledEnum"=T8."Enabled" ("Disabled")) -> ()  [unwired: 2 in, 2 out]
                    n3361 = property on="# of frames" class="DigNum (strict)"("DisabledEnum"=T8."Enabled" ("Disabled")) -> ()  [unwired: 2 in, 2 out]
                    n3362 = property on="save\ndata" class="Bool (strict)"("Value"=TRUE ("save\ndata")) -> ()  [unwired: 2 in, 2 out]
                  }
                  frame True {
                    w6543 = FALSE ("finite samples for recording")
                    n3363 = property on="finite samples" class="Bool (strict)"("Value"=w6543) -> ()  [unwired: 2 in, 2 out]
                    n3364 = property on="continuous" class="Bool (strict)"("Value"=w6543) -> ()  [unwired: 2 in, 2 out]
                    n3365 = property on="save\ndata" class="Bool (strict)"("DisabledEnum"=T8."Enabled" ("Disabled")) -> ()  [unwired: 2 in, 2 out]
                    n3366 = local write "Save tab"(enum32{"withsave", "withoutsave"}."withsave" ("Save tab")) -> ()
                    n3367 = property on="# of frames" class="DigNum (strict)"("DisabledEnum"=T8."Disabled" ("Disabled")) -> ()  [unwired: 2 in, 2 out]
                    n3368 = property on="save\ndata" class="Bool (strict)"("Value"=TRUE ("save\ndata")) -> ()  [unwired: 2 in, 2 out]
                  }
                }
              }
              frame #1 {
                n3369 = local read "finite samples"() -> (w6546:bool)
                n3370 = local read "continuous"() -> (w6547:bool)
                n3371 = local read "wavdet"() -> (w6548:bool)
                n3372 = call "2pparameters.vi"("command"="get") -> ("params out"=w6552:T12)  [unwired: 1 in]
                n3373 = Bundle By Name(cluster=w6552, "finite"=w6546, "cont"=w6547, "wavdet"=w6548) -> (w6549:T12)
                n3374 = call "2pparameters.vi"("Params in"=w6549, "command"="set") -> ()  [unwired: 1 out]
              }
            }
          }
          event "cursors": Value Change {
            n3375 = event-data() -> ()  [unwired: 1 in, 5 out]
            n3376 = case shown="True" "cursors" {
              frame False {
                n3377 = property on="img_CH1" class="IntGraph (strict)"("Active Cursor"=u32 0, "Cursor.Cursor Style"=u8 0 ("Cursor Style"), "Cursor.Cursor Point Style"=u8 0 ("Cursor Point Style")) -> ("Cursor.Cursor Position:Cursor X"=w6557:dbl, "Cursor.Cursor Position:Cursor Y"=w6558:dbl)  [unwired: 2 in, 2 out]
                n3378 = property on="img_CH2" class="IntGraph (strict)"("Active Cursor"=u32 0, "Cursor.Cursor Style"=u8 0 ("Cursor Style"), "Cursor.Cursor Point Style"=u8 0 ("Cursor Point Style")) -> ()  [unwired: 2 in, 2 out]
                n3379 = local write "cursor x [pixel]"(w6557) -> ()
                n3380 = local write "cursor y [pixel]"(w6558) -> ()
              }
              frame True {
                n3381 = stacked-sequence {
                  frame #0 {
                    n3382 = call "2pparameters.vi"("command"="get") -> ("params out"=w6573:T12)  [unwired: 1 in]
                    n3383 = Unbundle By Name(w6573) -> ("Xpixels Img"=w6574:i32, "Ypixels Img"=w6571:i32)
                    n3384 = To Double Precision Float(number=w6571) -> (double precision float=w6565:dbl)
                    n3385 = To Double Precision Float(number=w6574) -> (double precision float=w6570:dbl)
                    n3386 = Divide(x=w6565, y=2.0) -> (x/y=w6566:dbl)
                    n3387 = Divide(x=w6570, y=2.0) -> (x/y=w6568:dbl)
                    n3388 = Round To Nearest(number=w6566) -> (nearest integer value=w6564:dbl)
                    n3389 = Round To Nearest(number=w6568) -> (nearest integer value=w6567:dbl)
                    n3390 = property on="img_CH1" class="IntGraph (strict)"("Active Cursor"=u32 0, "Cursor.Cursor Style"=u8 8 ("Cursor Style"), "Cursor.Cursor Point Style"=u8 5 ("Cursor Point Style"), "Cursor.Cursor Position:Cursor X"=w6567, "Cursor.Cursor Position:Cursor Y"=w6564, "Cursor.Visible"=TRUE) -> ()  [unwired: 2 in, 2 out]
                  }
                  frame #1 {
                    n3391 = call "2pparameters.vi"("command"="get") -> ("params out"=w6593:T12)  [unwired: 1 in]
                    n3392 = call "2pparameters.vi"("command"="get") -> ("params out"=w6591:T12)  [unwired: 1 in]
                    n3393 = property on="img_CH1" class="IntGraph (strict)"("Active Cursor"=u32 0, "Cursor.Cursor Style"=u8 8 ("Cursor Style"), "Cursor.Cursor Point Style"=u8 5 ("Cursor Point Style")) -> ("Cursor.Cursor Position:Cursor X"=w6586:dbl, "Cursor.Cursor Position:Cursor Y"=w6585:dbl, "Cursor.Cursor Index"=w6608:i32, "Cursor.Cursor Plot"=w6607:i32, "Cursor.Visible"=w6578:bool)  [unwired: 2 in, 2 out]
                    "cursor x [pixel]" <- w6586
                    "cursor y [pixel]" <- w6585
                    n3394 = Unbundle By Name(w6593) -> ("Vy-max Img"=w6595:dbl, "Vy-min Img"=w6582:dbl, "Ypixels Img"=w6597:i32)
                    n3395 = Unbundle By Name(w6591) -> ("VX-max Img"=w6592:dbl, "Vx-min Img"=w6580:dbl, "Xpixels Img"=w6596:i32)
                    n3396 = Subtract(x=w6595, y=w6582) -> (x-y=w6600:dbl)
                    n3397 = Subtract(x=w6592, y=w6580) -> (x-y=w6598:dbl)
                    n3398 = local read "img_CH2"() -> (w6604:sgl[][])
                    n3399 = To Double Precision Float(number=w6596) -> (double precision float=w6599:dbl)
                    n3400 = local read "img_CH1"() -> (w6605:sgl[][])
                    n3401 = To Double Precision Float(number=w6597) -> (double precision float=w6601:dbl)
                    n3402 = Index Array(array=w6605, index (row)=w6608, index (col)=w6607) -> (element=→"value CH 1":sgl)
                    n3403 = Index Array(array=w6604, index (row)=w6608, index (col)=w6607) -> (element=→"value CH 2":sgl)
                    n3404 = Divide(x=w6598, y=w6599) -> (x/y=w6602:dbl)
                    n3405 = Divide(x=w6600, y=w6601) -> (x/y=w6603:dbl)
                    n3406 = Multiply(x=w6586, y=w6602) -> (x*y=w6581:dbl)
                    n3407 = Multiply(x=w6585, y=w6603) -> (x*y=w6584:dbl)
                    n3408 = property on="img_CH2" class="IntGraph (strict)"("Active Cursor"=u32 0, "Cursor.Cursor Style"=u8 8 ("Cursor Style"), "Cursor.Cursor Point Style"=u8 5 ("Cursor Point Style"), "Cursor.Cursor Position:Cursor X"=w6586, "Cursor.Cursor Position:Cursor Y"=w6585, "Cursor.Visible"=w6578) -> ()  [unwired: 2 in, 2 out]
                    n3409 = Add(x=w6581, y=w6580) -> (x+y=w6579:dbl)
                    n3410 = Add(x=w6584, y=w6582) -> (x+y=w6583:dbl)
                    n3411 = local write "Vx-ref"(w6579) -> ()
                    n3412 = local write "Vy-ref"(w6583) -> ()
                  }
                }
              }
            }
          }
          event "img_CH1": Cursor Move {
            n3413 = event-data() -> ("CursIdx"=w6613:i32)  [unwired: 1 in]
            n3414 = Equal To 0?(x=w6613) -> (x = 0?=w6614:bool)
            n3415 = case shown="True" w6614 {
              frame False {
              }
              frame True {
                n3416 = call "2pparameters.vi"("command"="get") -> ("params out"=w6634:T12)  [unwired: 1 in]
                n3417 = call "2pparameters.vi"("command"="get") -> ("params out"=w6636:T12)  [unwired: 1 in]
                n3418 = property on="img_CH1" class="IntGraph (strict)"("Active Cursor"=u32 0, "Cursor.Cursor Style"=u8 8 ("Cursor Style"), "Cursor.Cursor Point Style"=u8 5 ("Cursor Point Style")) -> ("Cursor.Cursor Position:Cursor X"=w6623:dbl, "Cursor.Cursor Position:Cursor Y"=w6622:dbl, "Cursor.Cursor Plot"=w6642:i32, "Cursor.Cursor Index"=w6641:i32, "Cursor.Visible"=w6615:bool)  [unwired: 2 in, 2 out]
                n3419 = Unbundle By Name(w6634) -> ("Vy-max Img"=w6632:dbl, "Vy-min Img"=w6621:dbl, "Ypixels Img"=w6630:i32)
                n3420 = Unbundle By Name(w6636) -> ("VX-max Img"=w6635:dbl, "Vx-min Img"=w6616:dbl, "Xpixels Img"=w6631:i32)
                n3421 = Subtract(x=w6632, y=w6621) -> (x-y=w6627:dbl)
                n3422 = Subtract(x=w6635, y=w6616) -> (x-y=w6629:dbl)
                n3423 = local write "cursor x [pixel]"(w6623) -> ()
                n3424 = local write "cursor y [pixel]"(w6622) -> ()
                n3425 = To Double Precision Float(number=w6631) -> (double precision float=w6628:dbl)
                n3426 = To Double Precision Float(number=w6630) -> (double precision float=w6626:dbl)
                n3427 = local read "img_CH2"() -> (w6643:sgl[][])
                n3428 = local read "img_CH1"() -> (w6646:sgl[][])
                n3429 = Index Array(array=w6643, index (row)=w6642, index (col)=w6641) -> (element=w6644:sgl)
                n3430 = Index Array(array=w6646, index (row)=w6642, index (col)=w6641) -> (element=w6645:sgl)
                n3431 = Divide(x=w6629, y=w6628) -> (x/y=w6625:dbl)
                n3432 = Divide(x=w6627, y=w6626) -> (x/y=w6624:dbl)
                n3433 = local write "value CH 2"(w6644) -> ()
                n3434 = Multiply(x=w6623, y=w6625) -> (x*y=w6618:dbl)
                n3435 = local write "value CH 1"(w6645) -> ()
                n3436 = Multiply(x=w6622, y=w6624) -> (x*y=w6620:dbl)
                n3437 = Add(x=w6618, y=w6616) -> (x+y=w6617:dbl)
                n3438 = local write "Vx-ref"(w6617) -> ()
                n3439 = Add(x=w6620, y=w6621) -> (x+y=w6619:dbl)
                n3440 = property on="img_CH2" class="IntGraph (strict)"("Active Cursor"=u32 0, "Cursor.Cursor Style"=u8 8 ("Cursor Style"), "Cursor.Cursor Point Style"=u8 5 ("Cursor Point Style"), "Cursor.Cursor Position:Cursor X"=w6623, "Cursor.Cursor Position:Cursor Y"=w6622, "Cursor.Visible"=w6615) -> ()  [unwired: 2 in, 2 out]
                n3441 = local write "Vy-ref"(w6619) -> ()
              }
            }
          }
          event "img_CH2": Cursor Move {
            n3442 = event-data() -> ("CursIdx"=w6650:i32)  [unwired: 1 in]
            n3443 = Equal To 0?(x=w6650) -> (x = 0?=w6651:bool)
            n3444 = case shown="True" w6651 {
              frame False {
              }
              frame True {
                n3445 = property on="img_CH2" class="IntGraph (strict)"("Active Cursor"=u32 0, "Cursor.Cursor Style"=u8 8 ("Cursor Style"), "Cursor.Cursor Point Style"=u8 5 ("Cursor Point Style")) -> ("Cursor.Cursor Position:Cursor X"=w6659:dbl, "Cursor.Cursor Position:Cursor Y"=w6660:dbl, "Cursor.Cursor Plot"=w6679:i32, "Cursor.Cursor Index"=w6678:i32, "Cursor.Visible"=w6652:bool)  [unwired: 2 in, 2 out]
                n3446 = call "2pparameters.vi"("command"="get") -> ("params out"=w6671:T12)  [unwired: 1 in]
                n3447 = call "2pparameters.vi"("command"="get") -> ("params out"=w6673:T12)  [unwired: 1 in]
                n3448 = local read "img_CH1"() -> (w6683:sgl[][])
                n3449 = local read "img_CH2"() -> (w6680:sgl[][])
                n3450 = local write "cursor x [pixel]"(w6659) -> ()
                n3451 = local write "cursor y [pixel]"(w6660) -> ()
                n3452 = Unbundle By Name(w6671) -> ("Vy-max Img"=w6669:dbl, "Vy-min Img"=w6654:dbl, "Ypixels Img"=w6667:i32)
                n3453 = Unbundle By Name(w6673) -> ("VX-max Img"=w6672:dbl, "Vx-min Img"=w6657:dbl, "Xpixels Img"=w6668:i32)
                n3454 = Index Array(array=w6683, index (row)=w6679, index (col)=w6678) -> (element=w6682:sgl)
                n3455 = Index Array(array=w6680, index (row)=w6679, index (col)=w6678) -> (element=w6681:sgl)
                n3456 = local write "value CH 2"(w6681) -> ()
                n3457 = local write "value CH 1"(w6682) -> ()
                n3458 = Subtract(x=w6669, y=w6654) -> (x-y=w6664:dbl)
                n3459 = Subtract(x=w6672, y=w6657) -> (x-y=w6666:dbl)
                n3460 = To Double Precision Float(number=w6668) -> (double precision float=w6665:dbl)
                n3461 = To Double Precision Float(number=w6667) -> (double precision float=w6663:dbl)
                n3462 = Divide(x=w6666, y=w6665) -> (x/y=w6662:dbl)
                n3463 = Divide(x=w6664, y=w6663) -> (x/y=w6661:dbl)
                n3464 = Multiply(x=w6659, y=w6662) -> (x*y=w6658:dbl)
                n3465 = Multiply(x=w6660, y=w6661) -> (x*y=w6655:dbl)
                n3466 = property on="img_CH1" class="IntGraph (strict)"("Active Cursor"=u32 0, "Cursor.Cursor Style"=u8 8 ("Cursor Style"), "Cursor.Cursor Point Style"=u8 5 ("Cursor Point Style"), "Cursor.Cursor Position:Cursor X"=w6659, "Cursor.Cursor Position:Cursor Y"=w6660, "Cursor.Visible"=w6652) -> ()  [unwired: 2 in, 2 out]
                n3467 = Add(x=w6658, y=w6657) -> (x+y=→"Vx-ref":dbl)
                n3468 = Add(x=w6655, y=w6654) -> (x+y=→"Vy-ref":dbl)
              }
            }
          }
          event "auto shutter": Value Change {
